vi "testWinX32Cam.vi"() -> ()   [LabVIEW 2011, in "run.lvlib"]
uses:
  run.lvlib
  Tools/Filing/FileSystem/FileSystem.lvclass
  Tools/CameraSettings/CamaraSettings.lvclass
  HWController/Network Controllers/NetworkCamera/NetworkCamera.lvclass
  Channels/Camera/WinX32_SA/WinX32Camera.lvclass
  Tools/Filing/FileNeologist/FileNeologist.lvclass
panel:
  out "stopped":bool
  in  "stop":bool
  out "error out":errorcluster
  in  "number":i32=1
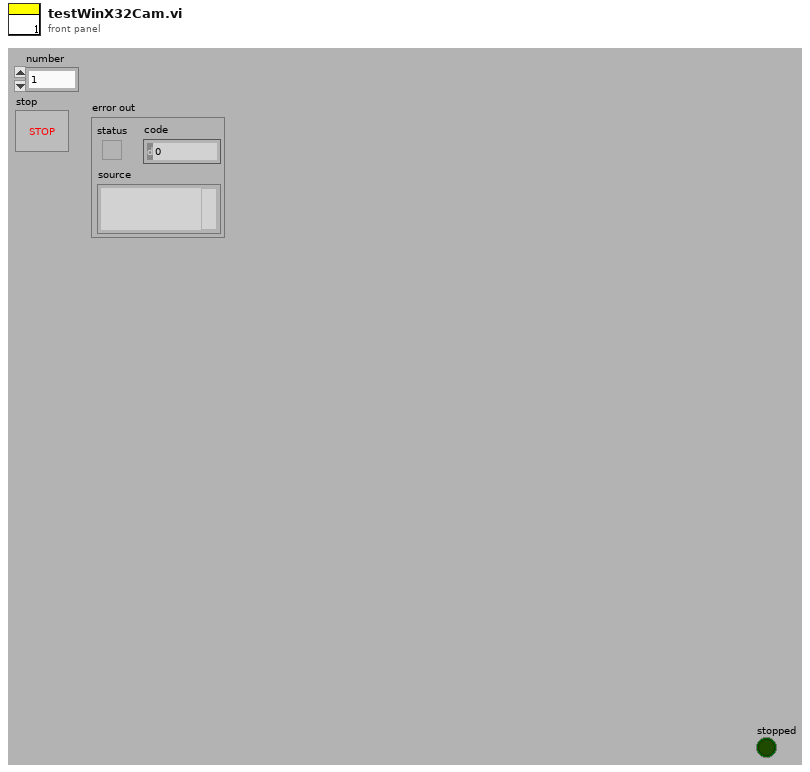
[diagram p1: front panel]
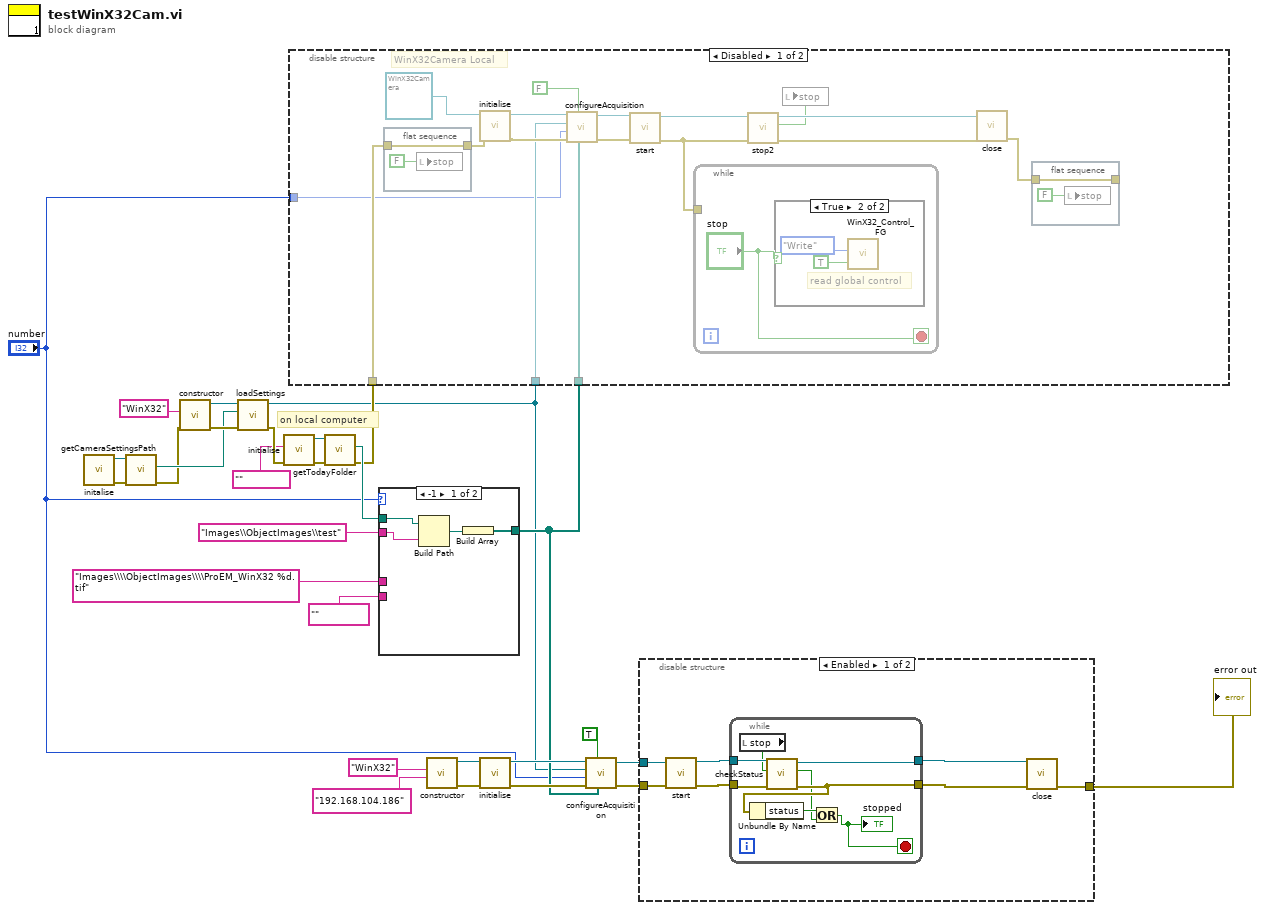
[diagram p0: block diagram]
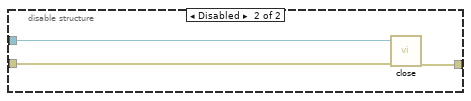
[diagram p2: hidden frame]
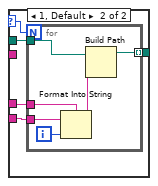
[diagram p5: hidden frame]
diagram:
  # "on local computer"
  n1 = call "initalise.vi"() -> ("error out"=w26:errorcluster, "FileSystem out"=w27:refnum<class "FileSystem.lvclass">)  [unwired: 10 in]
  n2 = call-dynamic "getCameraSettingsPath.vi"("error in (no error)"=w26, "FileSystem.lvclass in"=w27) -> ("error out"=w24:errorcluster, "CameraSettingsPath"=w25:path)  [unwired: 7 in, 1 out]
  n3 = call "constructor.vi"("error in (no error)"=w24, "camera settings"="WinX32" ("Camera")) -> ("error out"=w28:errorcluster, "CamaraSettings out"=w29:refnum<class "CamaraSettings.lvclass">)  [unwired: 8 in]
  n4 = call-dynamic "loadSettings.vi"("error in (no error)"=w28, "Path"=w25, "CamaraSettings in"=w29) -> ("error out"=w23:errorcluster, "CamaraSettings out"=w3:refnum<class "CamaraSettings.lvclass">)  [unwired: 7 in]
  n5 = call "initialise.vi"("error in (no error)"=w23, "computer name"="") -> ("error out"=w21:errorcluster, "FileNeologist out"=w22:refnum<class "FileNeologist.lvclass">)  [unwired: 8 in]
  n6 = call "getTodayFolder.vi"("error in (no error)"=w21, "FileNeologist in"=w22) -> ("error out"=w14:errorcluster, "todayFolder"=w19:path)  [unwired: 7 in, 1 out]
  n7 = case shown="-1" "number" {
    selector: "number" -> [_ w35]
    tunnel: w19 -> [w32 w38]
    tunnel: [w33 w37] -> w5
    tunnel: "Images\\\\ObjectImages\\\\ProEM_WinX32 %d.tif" -> [_ w36]
    tunnel: "" -> [_ w34]
    tunnel: "Images\\ObjectImages\\test" -> [w31 _]
    frame -1 {
      n8 = Build Path(base path=w32, name or relative path=w31) -> (appended path=w30:path)
      n9 = Build Array(w30) -> (w33:path[])
    }
    frame 1, Default {
      n10 = for {
        N: w35 -> [_]
        tunnel: w38 -> [w44]
        tunnel: [w43] -> w37 mode=indexing
        tunnel: w36 -> [w41]
        tunnel: w34 -> [w39]
        i -> [w42]
        n11 = Format Into String(format string=w41, initial string=w39, w42) -> (resulting string=w40:string)  [unwired: 1 in, 1 out]
        n12 = Build Path(base path=w44, name or relative path=w40) -> (appended path=w43:path)
      }
    }
  }
  n13 = disable-structure shown="Disabled" {
    disable-tunnel: w14 -> [w51 _]
    disable-tunnel: w5 -> [w47 _]
    disable-tunnel: w3 -> [w46 _]
    disable-tunnel: "number" -> [w45 _]
    frame Disabled {
      # "WinX32Camera Local"
      n14 = flat-sequence {
        tunnel: w51 -> [w65]
        tunnel: [w65] -> w50
        frame #0 {
          n15 = local write "stop"(FALSE ("stop")) -> ()
        }
      }
      n16 = call "initialise.vi"("error in (no error)"=w50, "WinX32Camera in"=refnum<class "WinX32Camera.lvclass"> refnum) -> ("error out"=w61:errorcluster, "WinX32Camera out"=w62:refnum<class "WinX32Camera.lvclass">)  [unwired: 8 in]
      n17 = call "configureAcquisition.vi"("imagePaths"=w47, "saveImages?"=FALSE, "error in (no error)"=w61, "number of Images"=w45, "CameraSettings"=w46, "WinX32Camera in"=w62) -> ("error out"=w57:errorcluster, "WinX32Camera out"=w58:refnum<class "WinX32Camera.lvclass">)  [unwired: 4 in]
      n18 = call "start.vi"("error in (no error)"=w57, "WinX32Camera in"=w58) -> ("error out"=w53:errorcluster, "WinX32Camera out"=w56:refnum<class "WinX32Camera.lvclass">)  [unwired: 8 in]
      n19 = while {
        tunnel: w53 -> [_]
        stop <- "stop" stop-if-true
        n20 = case shown="True" "stop" {
          frame False {
          }
          frame True {
            # "read global control"
            n21 = call "WinX32_Control_FG.vi"("stop"=TRUE, "Action"=enum16{"Write", "Read"}."Write") -> ()  [unwired: 9 in, 1 out]
          }
        }
      }
      n22 = call "stop2.vi"("error in (no error)"=w53, "WinX32Camera in"=w56) -> ("error out"=w54:errorcluster, "stopped?"=w52:bool, "WinX32Camera out"=w55:refnum<class "WinX32Camera.lvclass">)  [unwired: 6 in, 1 out]
      n23 = local write "stop"(w52) -> ()
      n24 = call "close.vi"("error in (no error)"=w54, "WinX32Camera in"=w55) -> ("error out"=w49:errorcluster)  [unwired: 8 in, 1 out]
      n25 = flat-sequence {
        tunnel: w49 -> [w63]
        tunnel: [w63] -> w48
        frame #0 {
          n26 = local write "stop"(FALSE ("stop")) -> ()
        }
      }
    }
    frame Enabled {
    }
  }
  n27 = call "constructor.vi"("machine name"="192.168.104.186", "Camera"="WinX32") -> ("error out"=w10:errorcluster, "NetworkCamera out"=w11:refnum<class "NetworkCamera.lvclass">)  [unwired: 8 in]
  n28 = call-dynamic "initialise.vi"("error in (no error)"=w10, "NetworkCamera in"=w11) -> ("error out"=w9:errorcluster, "NetworkCamera out"=w12:refnum<class "NetworkCamera.lvclass">)  [unwired: 8 in]
  n29 = call-dynamic "configureAcquisition.vi"("imagePaths"=w5, "saveImages?"=TRUE, "error in (no error)"=w9, "number of Images"="number", "CamaraSettings"=w3, "NetworkCamera in"=w12) -> ("error out"=w8:errorcluster, "NetworkCamera out"=w13:refnum<class "NetworkCamera.lvclass">)  [unwired: 4 in]
  n30 = disable-structure shown="Enabled" {
    disable-tunnel: w13 -> [w76 w85]
    disable-tunnel: w8 -> [w75 w86]
    disable-tunnel: [w70 w87] -> w1
    frame Enabled {
      n31 = call-dynamic "start.vi"("error in (no error)"=w75, "NetworkCamera in"=w76) -> ("error out"=w71:errorcluster, "NetworkCamera out"=w72:refnum<class "NetworkCamera.lvclass">)  [unwired: 8 in]
      n32 = while {
        tunnel: w72 -> [w82]
        tunnel: w71 -> [w81]
        tunnel: [w78] -> w74
        tunnel: [w79] -> w73
        stop <- w83 stop-if-true
        n33 = local read "stop"() -> (w80:bool)
        n34 = call-dynamic "checkStatus.vi"("error in (no error)"=w81, "stop"=w80, "NetworkCamera in"=w82) -> ("error out"=w79:errorcluster, "stopped?"=w77:bool, "NetworkCamera out"=w78:refnum<class "NetworkCamera.lvclass">)  [unwired: 6 in]
        n35 = Unbundle By Name(w79) -> ("status"=w84:bool)
        n36 = Or(x=w84, y=w77) -> (x .or. y?=w83:bool)
        "stopped" <- w83
      }
      n37 = call-dynamic "close.vi"("error in (no error)"=w73, "NetworkCamera in"=w74) -> ("error out"=w70:errorcluster)  [unwired: 9 in]
    }
    frame Disabled {
      n38 = call-dynamic "close.vi"("error in (no error)"=w86, "NetworkCamera in"=w85) -> ("error out"=w87:errorcluster)  [unwired: 9 in]
    }
  }
  "error out" <- w1
